vi "TX DRAM generation throughut test.vi"() -> ()   [LabVIEW 2019]
uses:
  SubVIs/DRAM burst sequencer/SegementSequencer_class/FPGA sequencer states.ctl
  SubVIs/DRAM burst sequencer/DRAM mode.ctl
  <vilib>/Platform/TimedLoop/XDataNode/timing_clust.ctl
  <vilib>/Platform/TimedLoop/XDataNode/nitl_modes.ctl
  <vilib>/Platform/TimedLoop/XDataNode/wakeup.ctl
  SubVIs/DRAM burst sequencer/DRAM resources.ctl
  <instrlib>/_niInstr/Memory/v1/FPGA/DRAM U512/niInstr Memory DRAM U512 v1 FPGA.lvclass
  <instrlib>/_niInstr/Memory/v1/FPGA/BRAM U512/niInstr Memory BRAM U512 v1 FPGA.lvclass
  <instrlib>/_niInstr/Memory/v1/FPGA/DRAM U512/Public/Create.vi
  <vilib>/rvi/DataTransferAndStorage/Container/Common/niFpgaContainerGetUniqueNameForEmu.vi
  <vilib>/rvi/DataTransferAndStorage/Container/Common/niFpgaContainerSetEmuInfo.vi
  <vilib>/rvi/eio/common/nirviEmuReportErrorAndStop.vi
  <vilib>/rvi/Emulation/niFpgaSctlEmulationGetInTimedLoop.vi
  <vilib>/rvi/Emulation/niFpgaEmulationReportErrorSimple.vi
  <vilib>/rvi/Emulation/niFpgaGetClockAttributes.vi
  <vilib>/rvi/Emulation/niFpgaCriticalErrorInLSC.vi
  <vilib>/rvi/Emulation/niFpgaProcessEmulError.vi
  <instrlib>/_niInstr/Basic Elements/v1/FPGA/Private/Count Up U64.vi
  <vilib>/rvi/interface/RandomDataEmulation/nirviRandomDataMultiElementFPGAFIFO.vi
  <instcachedir>/0/nirviRandomDataMultiElementFPGAFIFO_1ED88BA00AC641F388A9B1FAA20E354D.lvgen/nirviRandomDataMultiElementFPGAFIFO_1ED88BA00AC641F388A9B1FAA20E354D_003.vi
  <vilib>/rvi/interface/RandomDataEmulation/niFpgaRandomDataHandleErrors.vi
  <instrlib>/_niInstr/Basic Elements/v1/FPGA/Private/Count Up U32.vi
  <vilib>/rvi/DataTransferAndStorage/Container/Common/niFpgaContainerExecOnDevCompGetState.vi
  <vilib>/rvi/Emulation/niFpgaEmulationIsFPGAContextNoSignature.vi
  <vilib>/rvi/errors/niFpgaSetErrorForExecOnDevCompSimple.vi
  <vilib>/rvi/FIFO/Fifo_Resource/nirvififoEmulationSetSize.vi
  <vilib>/rvi/FIFO/Fifo_Resource/nirviFifoEmulationQueueMgr.vi
  <instcachedir>/0/nirviFifoEmulationQueueMgr_E5CAEC123FF24DC58D834DCA3CDAA9B5.lvgen/nirviFifoEmulationQueueMgr_E5CAEC123FF24DC58D834DCA3CDAA9B5_011.vi
  <vilib>/rvi/FIFO/Fifo_Resource/nirvififoEmulationDetermineInputValidOut.vi
  <vilib>/rvi/FIFO/Fifo_Resource/nirvififoEmulationCreateLock.vi
  <vilib>/rvi/FIFO/Fifo_Resource/nirvififoEmulationObtainLock.vi
  <vilib>/rvi/FIFO/Fifo_Resource/nirvififoEmulationReleaseLock.vi
  <vilib>/rvi/occurrence/nirviWaitOnOccurrenceBase.vi
  <vilib>/rvi/errors/nirviReportUnexpectedCaseInternalError.vi
  <vilib>/rvi/errors/nirviReportUnexpectedCaseInternalError (U32).vi
  <vilib>/Utility/error.llb/Clear Errors.vi
  <vilib>/platform/TimedLoop/XDataNode/XDataNode.xnode
  <vilib>/rvi/LocalResourceManager/LocalResourceManager.xnode
  <vilib>/rvi/DataTransferAndStorage/Container/XNode/niFpgaContainer.xnode
  <vilib>/rvi/interface/RandomDataEmulation/nirviRandomDataFpgaMultiElementTemplate.vi
  <vilib>/rvi/FIFO/Fifo_Resource/niFpgaFifoEmulationRefIn.vi
  SubVIs/DRAM burst sequencer/SegementSequencer_class/SegmentSequencer.lvclass
  <vilib>/Platform/TimedLoop/XDataNode/XDNodeRunTimeDep.lvlib
  <instrlib>/_niInstr/Memory/v1/FPGA/DRAM/niInstr Memory DRAM v1 FPGA.lvclass
  <instrlib>/_niInstr/Basic Elements/v1/FPGA/niInstr Basic Elements v1 FPGA.lvlib
  SubVIs/Utility/FPGA Utility.lvlib
  SubVIs/DRAM burst sequencer/TX burst sequencer.lvlib
panel:
  in  "dram mode":T1
  out "dram.debug ctr":T2
  in  "seq.continous":bool
  in  "debug end":u64
  in  "debug start":u64
  in  "dram.ctr rst":bool
  out "gen.pending to read":u32
  out "seq.req ctr":i64
  out "dram.last written addr":u32
  out "dma overflow":bool
  out "missed sample count":u32
  in  "gen.length":u64
  in  "gen.start":bool
  out "seq.loaded steps":u32
  out "seq.repeat ctr":u64
  out "seq.step ctr":u32
  out "seq.state":T3
  in  "seq.rst":bool
  in  "seq.start":bool
  in  "seq.new step":T4
  in  "seq.add step":bool
  in  "iq.load addr":u32
  in  "iq.load":bool
  in  "dram.reset":bool
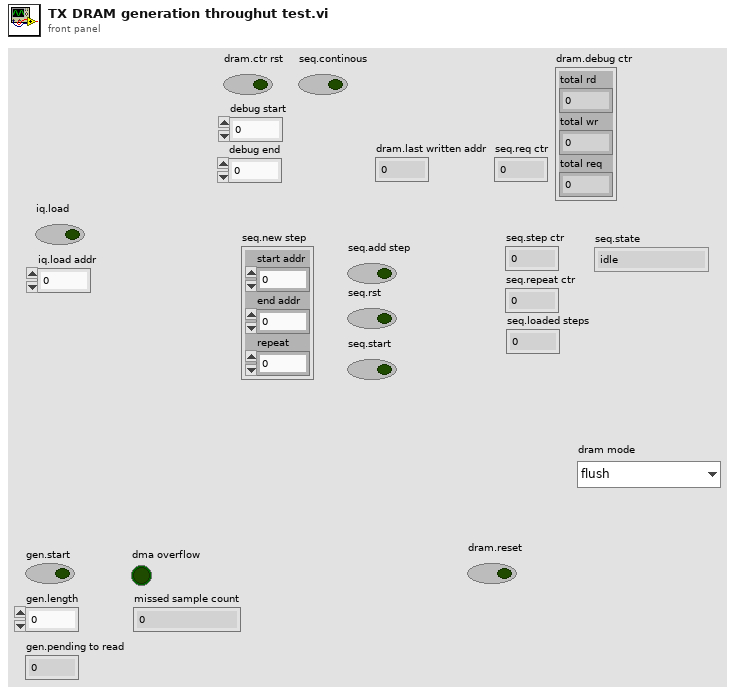
[diagram p1: front panel]
types:
  T1 = typedef "TX burst sequencer.lvlib/DRAM mode.ctl" = enum16{"flush", "reset", "write", "read"}
  T2 = cluster{"total rd":u32, "total wr":u32, "total req":u32}
  T3 = typedef "FPGA sequencer states.ctl" = enum16{"idle", "read step", "execute step"}
  T4 = cluster{"start addr":u32, "end addr":u32, "repeat":u64}
  T5 = typedef "TX burst sequencer.lvlib/DRAM resources.ctl" = cluster{"DRAM read data FIFO":refnum<k21>, "DRAM write data FIFO":refnum<k21>, "DRAM request FIFO":refnum<k21>, "DRAM U512 memo":refnum<class "niInstr Memory DRAM U512 v1 FPGA.lvclass">, "DMA data loader":refnum<k21>, "BRAM read data FIFO":refnum<k21>, "BRAM write data FIFO":refnum<k21>, "BRAM request FIFO":refnum<k21>, "BRAM U512 memo":refnum<class "niInstr Memory BRAM U512 v1 FPGA.lvclass">}
  T6 = typedef "XDNodeRunTimeDep.lvlib/timing_clust.ctl" = cluster{"Expected End [f-1]":u64, "Actual End [f-1]":u64, "Finished Late? [f-1]":bool, "Expected End [i-1]":u64, "Actual End [i-1]":u64, "Finished Late? [i-1]":bool, "Expected Start [i]":u64, "Actual Start [i]":u64, "Expected Start [f]":u64, "Actual Start [f]":u64, "Source Name":string, "Structure Name":string, "Period":i64, "Deadline":i64, "Offset":i64, "Start":i64, "Priority":i32, "Timeout":i32, "Mode":T7, "Wakeup Reason":T8, "Error":errorcluster, "Source Type":string, "Secondary Source Type":string, "Global End Time":u64, "Global Start Time":u64, "Frame Duration":u64, "Iteration Duration":u64, "Assigned CPU":i32, "I/O Scan Engine Mode":u32}
  T7 = typedef "XDNodeRunTimeDep.lvlib/nitl_modes.ctl" = enum32{"No Change", "Process missed periods, maintain original phase", "Discard missed periods, maintain original phase", "Process missed periods, ignore original phase", "Discard missed periods, ignore original phase"}
  T8 = typedef "XDNodeRunTimeDep.lvlib/wakeup.ctl" = enum32{"Normal", "Aborted", "Asynchronous wakeup", "Timing source error", "Timed loop error", "Timeout"}
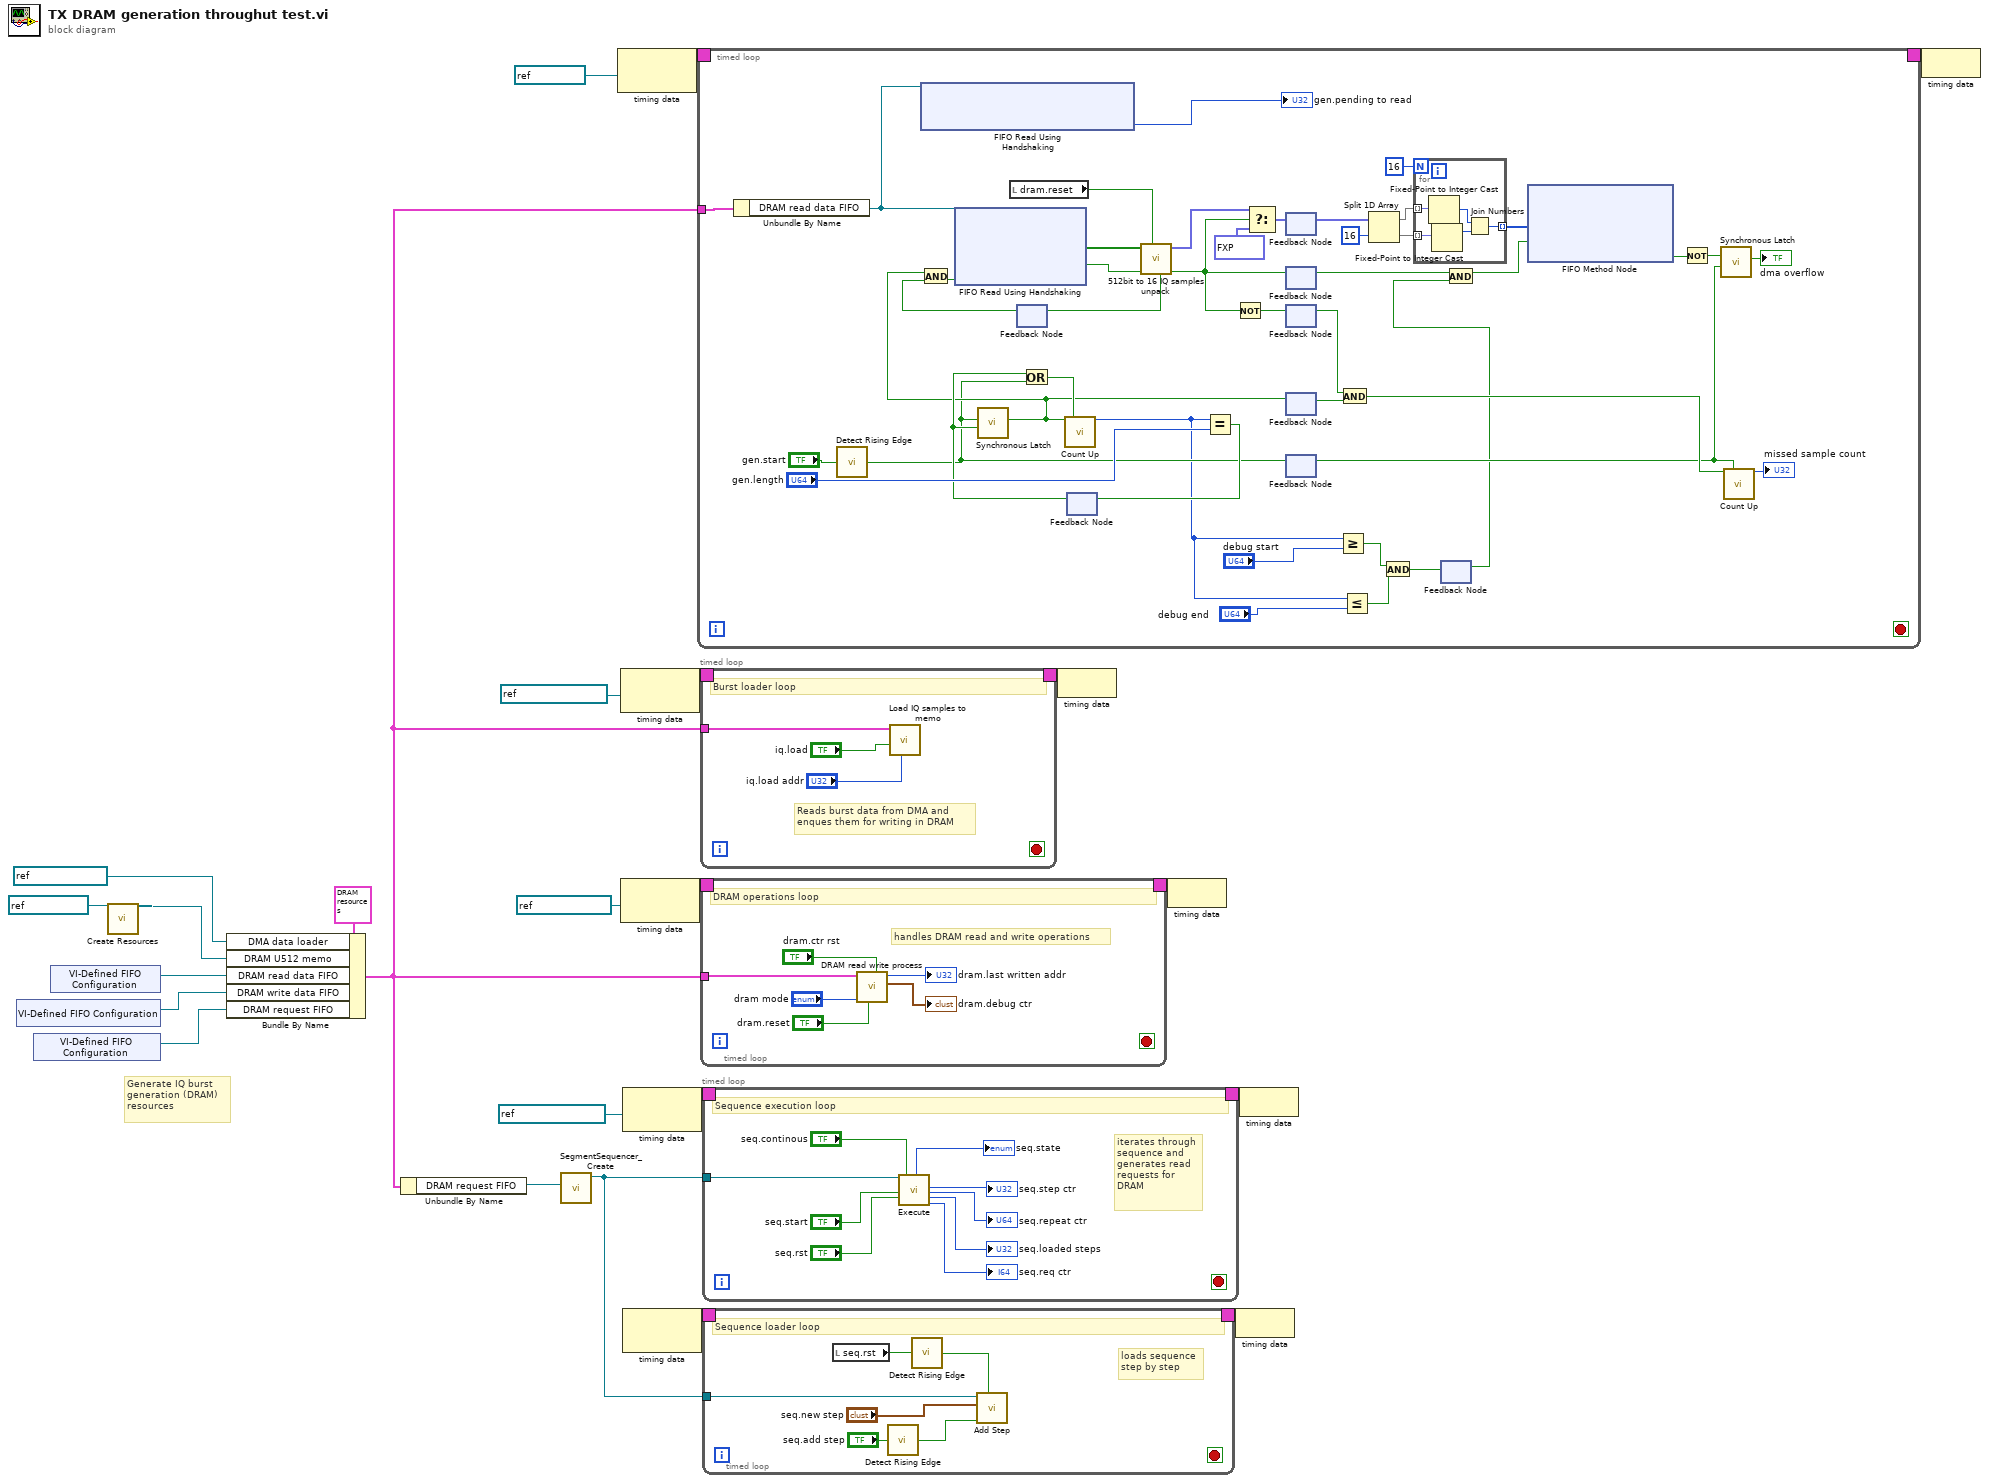
[diagram p0: block diagram]
diagram:
  # "Generate IQ burst\ngeneration (DRAM)\nresources"
  n1 = xnode "VI-Defined FIFO Configuration"() -> ("FIFO Out"=w6:refnum<k21>)
  n2 = xnode "VI-Defined FIFO Configuration"() -> ("FIFO Out"=w5:refnum<k21>)
  n3 = xnode "VI-Defined FIFO Configuration"() -> ("FIFO Out"=w7:refnum<k21>)
  n4 = call-poly <instrlib>:"Create Resources.vi"("memory in"=refnum<k21> "TX memo") -> ("memory out"=w4:refnum<class "niInstr Memory DRAM U512 v1 FPGA.lvclass">)  [unwired: 14 in]
  n5 = Bundle By Name(cluster=T5 {"DRAM read data FIFO"="", "DRAM write data FIFO"="", "DRAM request FIFO"="", "DRAM U512 memo"=refnum, "DMA data loader"="custom data", "BRAM read data FIFO"="", "BRAM write data FIFO"="", "BRAM request FIFO"="", "BRAM U512 memo"=refnum} ("DRAM resources"), "DMA data loader"=refnum<k21> "custom data" ("FIFO In"), "DRAM U512 memo"=w4, "DRAM read data FIFO"=w7, "DRAM write data FIFO"=w6, "DRAM request FIFO"=w5) -> (w2:T5)
  n6 = Unbundle By Name(w2) -> ("DRAM request FIFO"=w1:refnum<k21>)
  n7 = call "SegmentSequencer_Create.vi"("req fifo 2"=w1) -> ("New SegmentSequencer"=w12:refnum<class "SegmentSequencer.lvclass">)  [unwired: 10 in]
  n8 = node-c288(refnum<k21> "192MHz" ("Source Name")) -> (w11:T6)
  n9 = node-c288(refnum<k21> "100 MHz Clock" ("Source Name")) -> (w20:T6)
  n10 = node-c288(refnum<k21> "DRAM Clock" ("Source Name")) -> (w24:T6)
  n11 = node-c288(refnum<k21> "200 MHz Clock" ("Source Name")) -> (w15:T6)
  n12 = node-c288() -> (w17:T6)  [unwired: 1 in]
  n13 = timed-loop {
    timing: w11 -> [_]
    timing-out: [_] -> w10
    tunnel: w2 -> [w26]
    stop <- _ stop-if-true
    n14 = Unbundle By Name(w26) -> ("DRAM read data FIFO"=w25:refnum<k21>)
    n15 = call <instrlib>:"Detect Rising Edge.vi"("signal"="gen.start") -> ("edge detected"=w39:bool)  [unwired: 14 in]
    n16 = xnode ("FIFO Read Using Handshaking")("FIFO In"=w25) -> ("Number of Elements to Read"=→"gen.pending to read":u32)  [unwired: 1 out]
    n17 = local read "dram.reset"() -> (w41:bool)
    n18 = feedback #1() -> (w65:bool)  [unwired: 1 in]
    n19 = feedback #2() -> (w59:bool)  [unwired: 1 in]
    n20 = call <instrlib>:"Synchronous Latch.vi"("clear"=w59, "set"=w39) -> ("out"=w58:bool)  [unwired: 9 in]
    n21 = And(x=w58, y=w65) -> (x .and. y?=w64:bool)
    n22 = xnode ("FIFO Read Using Handshaking")("Ready for Output"=w64, "FIFO In"=w25) -> ("Element"=w68:bool[], "Output Valid"=w67:bool)  [unwired: 1 out]
    n23 = Or(x=w59, y=w39) -> (x .or. y?=w61:bool)
    n24 = call-poly <instrlib>:"Count Up.vi"("increment"=w58, "reset"=w61) -> ("count out"=w37:u64)  [unwired: 13 in]
    n25 = call "512bit to 16 IQ samples unpack.vi"("reset"=w41, "input valid"=w67, "data in"=w68) -> ("output valid"=w30:bool, "data out"=w29:fxp<+/-,12,1>[], "ready for input"=w66:bool)  [unwired: 6 in]
    n26 = feedback-in #1(w66) -> ()
    n27 = Equal?(x=w37, y="gen.length") -> (x = y?=w60:bool)
    n28 = feedback-in #2(w60) -> ()
    n29 = Not(x=w30) -> (.not. x?=w57:bool)
    n30 = Select(t=w29, s=w30, f=fxp<+/-,12,1>[] [0.0, 0.0, 0.0, 0.0, 0.0, 0.0, 0.0, 0.0, 0.0, 0.0, 0.0, 0.0, 0.0, 0.0, 0.0, 0.0, 0.0, 0.0, 0.0, 0.0, 0.0, 0.0, 0.0, 0.0, 0.0, 0.0, 0.0, 0.0, 0.0, 0.0, 0.0, 0.0] ("data out")) -> (s? t:f=w28:fxp<+/-,12,1>[])
    n31 = feedback #3() -> (w52:fxp<+/-,12,1>[])  [unwired: 1 in]
    n32 = feedback-in #3(w28) -> ()
    n33 = feedback #4() -> (w46:bool)  [unwired: 1 in]
    n34 = feedback-in #4(w30) -> ()
    n35 = feedback-in #5(w57) -> ()
    n36 = feedback #5() -> (w55:bool)  [unwired: 1 in]
    n37 = feedback-in #6(w58) -> ()
    n38 = feedback #6() -> (w54:bool)  [unwired: 1 in]
    n39 = feedback #7() -> (w42:bool)  [unwired: 1 in]
    n40 = feedback-in #7(w39) -> ()
    n41 = Greater Or Equal?(x=w37, y="debug start") -> (x >= y?=w35:bool)
    n42 = And(x=w55, y=w54) -> (x .and. y?=w56:bool)
    n43 = Less Or Equal?(x=w37, y="debug end") -> (x <= y?=w34:bool)
    n44 = Split 1D Array(array=w52, index=16) -> (first subarray=w50:fxp<+/-,12,1>[], second subarray=w49:fxp<+/-,12,1>[])
    n45 = And(x=w35, y=w34) -> (x .and. y?=w33:bool)
    n46 = for {
      N: 16 -> [_]
      tunnel: w50 -> [w73] mode=indexing
      tunnel: w49 -> [w71] mode=indexing
      tunnel: [w69] -> w47 mode=indexing
      n47 = Fixed-Point to Integer Cast(1:w73) -> (0:w72:i16)
      n48 = Fixed-Point to Integer Cast(1:w71) -> (0:w70:i16)
      n49 = Join Numbers(hi=w72, lo=w70) -> ((hi.lo)=w69:u32)
    }
    n50 = feedback #8() -> (w31:bool)  [unwired: 1 in]
    n51 = feedback-in #8(w33) -> ()
    n52 = And(x=w46, y=w31) -> (x .and. y?=w32:bool)
    n53 = xnode ("FIFO Method Node")("Element"=w47, "Input Valid"=w32) -> ("Ready for Input"=w45:bool)  [unwired: 1 in, 1 out]
    n54 = Not(x=w45) -> (.not. x?=w44:bool)
    n55 = call <instrlib>:"Synchronous Latch.vi"("clear"=w42, "set"=w44) -> ("out"=→"dma overflow":bool)  [unwired: 9 in]
    n56 = call-poly <instrlib>:"Count Up.vi"("increment"=w56, "reset"=w42) -> ("count out"=→"missed sample count":u32)  [unwired: 13 in]
  }
  n57 = timed-loop {
    timing: w20 -> [_]
    timing-out: [_] -> w19
    tunnel: w2 -> [w76]
    stop <- _ stop-if-true
    # "Reads burst data from DMA and\nenques them for writing in DRAM"
    # "Burst loader loop"
    n58 = call "Load IQ samples to memo.vi"("wr.start addr"="iq.load addr", "wr.enable"="iq.load", "DRAM resources"=w76) -> ()  [unwired: 9 in]
  }
  n59 = timed-loop {
    timing: w24 -> [_]
    timing-out: [_] -> w23
    tunnel: w2 -> [w82]
    stop <- _ stop-if-true
    # "handles DRAM read and write operations"
    # "DRAM operations loop"
    n60 = call "DRAM read write process.vi"("debug ctr reset"="dram.ctr rst", "dram.reset"="dram.reset", "dram mode"="dram mode", "DRAM resources"=w82) -> ("DRAM debug ctr"=→"dram.debug ctr":T2, "last written addr"=→"dram.last written addr":u32)  [unwired: 6 in]
  }
  n61 = timed-loop {
    timing: w15 -> [_]
    timing-out: [_] -> w14
    tunnel: w12 -> [w91]
    stop <- _ stop-if-true
    # "iterates through\nsequence and\ngenerates read\nrequests for\nDRAM"
    # "Sequence execution loop"
    n62 = call-dynamic "Execute.vi"("SegmentSequencer in"=w91, "start"="seq.start", "reset"="seq.rst", "continuous?"="seq.continous") -> ("state"=→"seq.state":T3, "step counter"=→"seq.step ctr":u32, "repeat counter"=→"seq.repeat ctr":u64, "Loaded steps"=→"seq.loaded steps":u32, "generated requests"=→"seq.req ctr":i64)  [unwired: 10 in, 1 out]
  }
  n63 = timed-loop {
    timing: w17 -> [_]
    timing-out: [_] -> w16
    tunnel: w12 -> [w105]
    stop <- _ stop-if-true
    # "loads sequence\nstep by step"
    # "Sequence loader loop"
    n64 = local read "seq.rst"() -> (w101:bool)
    n65 = call <instrlib>:"Detect Rising Edge.vi"("signal"="seq.add step") -> ("edge detected"=w104:bool)  [unwired: 14 in]
    n66 = call <instrlib>:"Detect Rising Edge.vi"("signal"=w101) -> ("edge detected"=w100:bool)  [unwired: 14 in]
    n67 = call-dynamic "Add Step.vi"("reset load"=w100, "input valid"=w104, "Data"="seq.new step", "SegmentSequencer in"=w105) -> ()  [unwired: 7 in, 1 out]
  }
  n68 = node-c288(w19) -> ()
  n69 = node-c288(w23) -> ()
  n70 = node-c288(w16) -> ()
  n71 = node-c288(w14) -> ()
  n72 = node-c288(w10) -> ()
